vi "to string array.vi"(8 "error in (no error)":errorcluster, 11 "Multiplexer configuration in":refnum<class "Multiplexer configuration.lvclass">) -> (0 "error out":errorcluster, 1 "Array":string[][](array[string]), 2 "version":string, 3 "Multiplexer configuration out":refnum<class "Multiplexer configuration.lvclass">)   [LabVIEW 2021, in "Multiplexer configuration.lvclass"]
uses:
  Multiplexer configuration.lvclass
  current version.vi
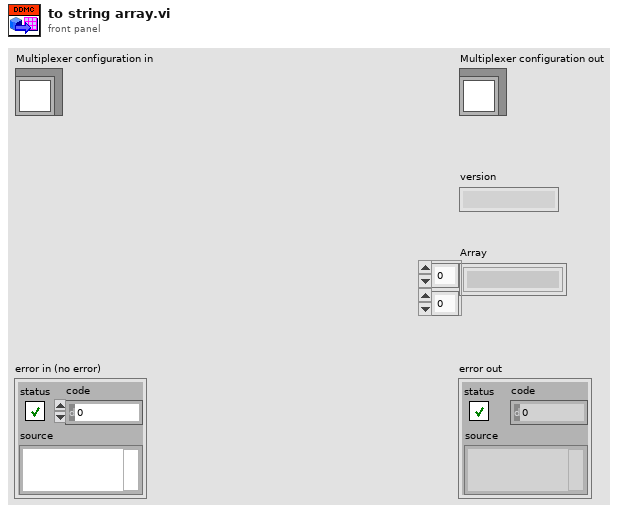
[diagram p1: front panel]
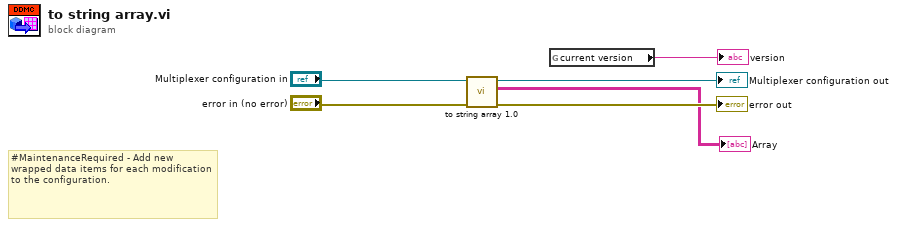
[diagram p0: block diagram]
diagram:
  # "#MaintenanceRequired - Add new wrapped data items for each modification to the configuration."
  n1 = call "to string array 1.0.vi"("error in (no error)"="error in (no error)", "Multiplexer configuration in"="Multiplexer configuration in") -> ("error out"=→"error out":errorcluster, "Array"=→"Array":string[][], "Multiplexer configuration out"=→"Multiplexer configuration out":refnum<class "Multiplexer configuration.lvclass">)  [unwired: 7 in]
  n2 = global read "current version.vi" "current version"() -> (→"version":string)
